vi "InitTimeStamp.vi"(8 "error in":errorcluster, 10 "Input Terminal":tag="/Dev3/10MHzRefClock", 11 "Counter":tag="Dev3/ctr1") -> (0 "error out":errorcluster, 3 "task out":refnum<k21>)   [LabVIEW 2014]
uses:
  <vilib>/DAQmx/create/channels.llb/DAQmx Create Channel (CI-Count Edges).vi
  <resource>/objmgr/daqmx.rc
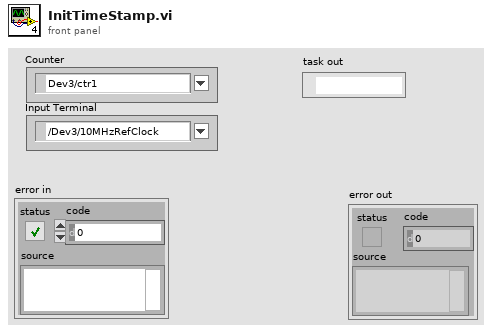
[diagram p1: front panel]
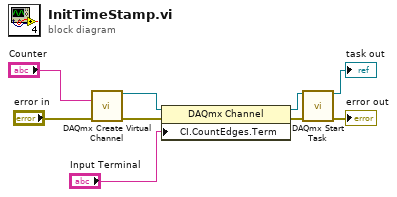
[diagram p0: block diagram]
diagram:
  n1 = call-poly <vilib>:"DAQmx Create Virtual Channel.vi"("counter"="Counter", "error in"="error in") -> ("task out"=w6:refnum<k21>, "error out"=w4:errorcluster)  [unwired: 12 in]
  n2 = property class="DAQmx Channel"(reference=w6, error in=w4, "CI.CountEdges.Term"="Input Terminal") -> (reference out=w9:refnum<k21>, error out=w8:errorcluster)
  n3 = call <vilib>:"DAQmx Start Task.vi"("task/channels in"=w9, "error in"=w8) -> ("task out"=→"task out":refnum<k21>, "error out"=→"error out":errorcluster)  [unwired: 12 in]
